vi "Test Error if Generating from Concrete Class.vi"(8 "error in (no error)":errorcluster, 11 "Test Case In":refnum<class "Responsive Mock Class Generator Test.lvclass">) -> (0 "error out":errorcluster, 3 "Test Case Out":refnum<class "Responsive Mock Class Generator Test.lvclass">)   [LabVIEW 2020, in "Responsive Mock Class Generator Test.lvclass"]
uses:
  Responsive Mock Class Generator Test.lvclass
  C:/Program Files (x86)/National Instruments/LabVIEW 2020/vi.lib/Astemes/LUnit/Test Case.lvclass
  <vilib>/Astemes/LUnit/Test Case.lvclass/Test Case.ctl
  <vilib>/Astemes/LUnit/Append Fail Result.vi
  <vilib>/Astemes/LUnit/Append Pass Result.vi
  source/Scripting/Mock Class Generator/Responsive Mock Class Generator.lvclass
  <vilib>/Astemes/LUnit/Test Case.lvclass
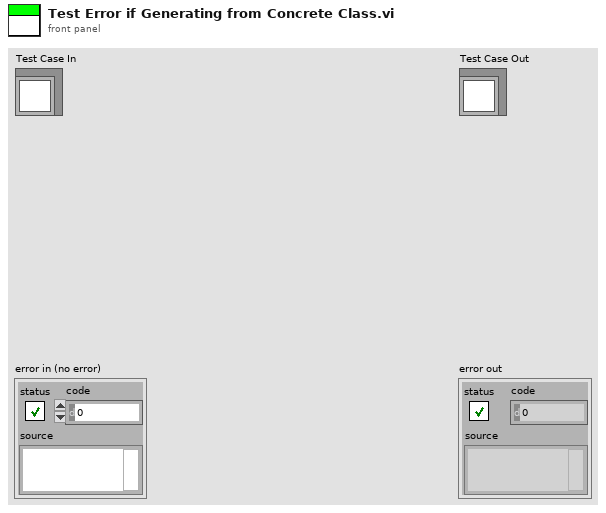
[diagram p1: front panel]
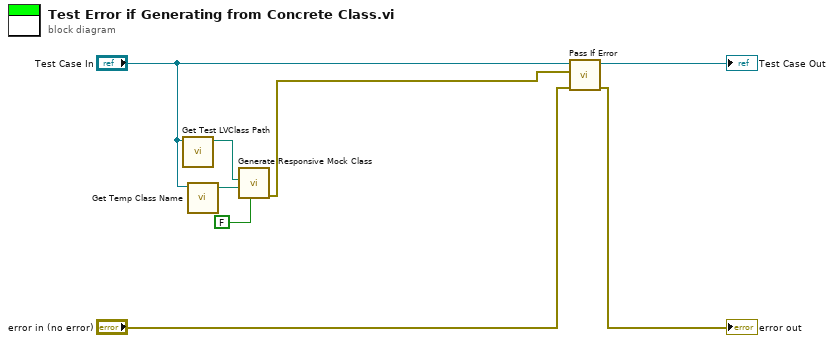
[diagram p0: block diagram]
diagram:
  n1 = call "Get Test LVClass Path.vi"("Mock Class Generator Test in"="Test Case In") -> ("Test Class Path"=w5:path)  [unwired: 10 in]
  n2 = call "Get Temp Class Name.vi"("Mock Class Generator Test in"="Test Case In") -> ("Test Class Path"=w3:path)  [unwired: 10 in]
  n3 = call "Generate Responsive Mock Class.vi"("Add to lvproj?"=FALSE, "Destination Class Path"=w3, "Source Class Path"=w5) -> ("error out"=w1:errorcluster)  [unwired: 8 in]
  n4 = call <vilib>:"Pass If Error.vi"("error in (no error)"="error in (no error)", "Assert error"=w1, "LUnit Test Case In"="Test Case In") -> ("error out"=→"error out":errorcluster, "LUnit Test Case Out"=→"Test Case Out":refnum<class "Responsive Mock Class Generator Test.lvclass">)  [unwired: 7 in]
